vi "add NI PSP Service Locator firewall.vi"() -> ()   [LabVIEW 2016]
uses:
  <vilib>/Utility/sysdir.llb/System Directory Type.ctl
  <vilib>/regexp/Match Regular Expression.xnode
panel:
  out "standard output":string caption="标准输出"
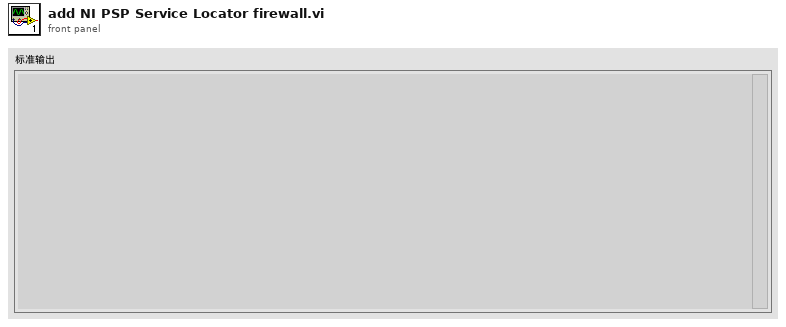
[diagram p1: front panel]
types:
  T1 = typedef "System Directory Type.ctl" = i32
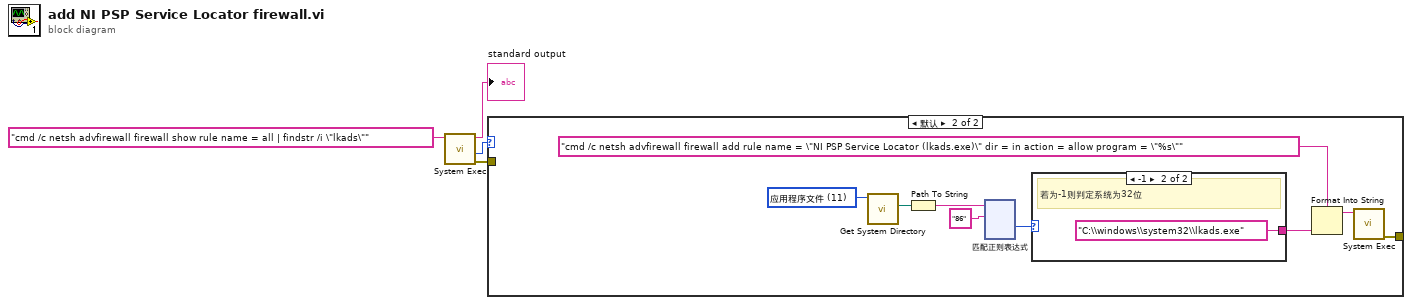
[diagram p0: block diagram]
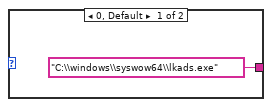
[diagram p3: hidden frame]
diagram:
  n1 = call <vilib>:"System Exec.vi"("command line"="cmd /c netsh advfirewall firewall show rule name = all | findstr /i \"lkads\"") -> ("error out"=w1:errorcluster, "return code"=w2:i32, "standard output"=→"standard output":string)  [unwired: 7 in, 1 out]
  n2 = case shown="默认" w2 {
    tunnel: w1 -> [_ _]
    tunnel: [_ w5] -> _
    frame 0 {
    }
    frame Default {
      w8 = T1 11 items=["用户目录"=0, "用户桌面"=1, "用户文档"=2, "用户应用程序数据"=3, "用户设置"=4, "用户临时目录"=5, "公共文档"=6, "公共应用程序数据"=7, "公共设置"=8, "公共缓存"=13, "系统核心库"=9, "系统安装库"=10, "应用程序文件"=11, "启动盘根目录"=12] ("system directory type")
      n3 = call <vilib>:"Get System Directory.vi"("system directory type"=w8) -> ("system directory"=w9:path)  [unwired: 10 in]
      n4 = Path To String(path=w9) -> (string=w10:string)
      n5 = xnode "匹配正则表达式"("输入字符串"=w10, "正则表达式"="86") -> ("匹配后偏移量"=w12:i32)  [unwired: 4 in, 4 out]
      n6 = case shown="-1" w12 {
        tunnel: ["C:\\windows\\syswow64\\lkads.exe" ("command line") "C:\\windows\\system32\\lkads.exe" ("command line")] -> w7
        frame 0, Default {
        }
        frame -1 {
          # "若为-1则判定系统为32位"
        }
      }
      n7 = Format Into String(format string="cmd /c netsh advfirewall firewall add rule name = \"NI PSP Service Locator (lkads.exe)\" dir = in action = allow program = \"%s\"" ("command line"), w7) -> (resulting string=w13:string)  [unwired: 2 in, 1 out]
      n8 = call <vilib>:"System Exec.vi"("command line"=w13) -> ("error out"=w5:errorcluster)  [unwired: 7 in, 3 out]
    }
  }
